vi "AO_2Chan.vi"() -> ()   [LabVIEW 2021]
doc: "This example demonstrates how to generate a user-defined voltage using the analog output of a DAQ device."
uses:
  <vilib>/Utility/error.llb/DialogType.ctl
  <vilib>/DAQmx/write.llb/DAQmx Write (Analog 1D DBL NChan 1Samp).vi
  <vilib>/DAQmx/create/channels.llb/DAQmx Create Channel (AO-Voltage-Basic).vi
  <vilib>/DAQmx/miscellaneous.llb/DAQmx Fill In Error Info.vi
panel:
  out "Iteration":i32
  in  "Tab Control":enum32{"Manual", "Toggle"}(tab)
  in  "Control":enum16{"Up", "Zero", "Down"}[](array[ring])
  out "Output":dbl[](array[numeric])
  in  "Pulse Width":u32=100
  in  "Stop":bool
  in  "Max Voltage":dbl=10.0
  in  "Min Voltage":dbl=-10.0
  in  "Physical Channel(s)":tag="Dev2/ao0:1"
  # "Channel Settings"
  # "Output"
  # "The number of elements in the channel array\nmust equal the number of channels in the task."
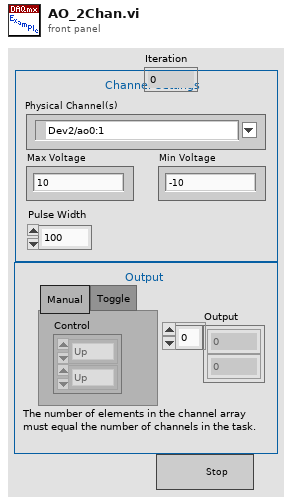
[diagram p1: front panel]
types:
  T1 = typedef "DialogType.ctl" = u16
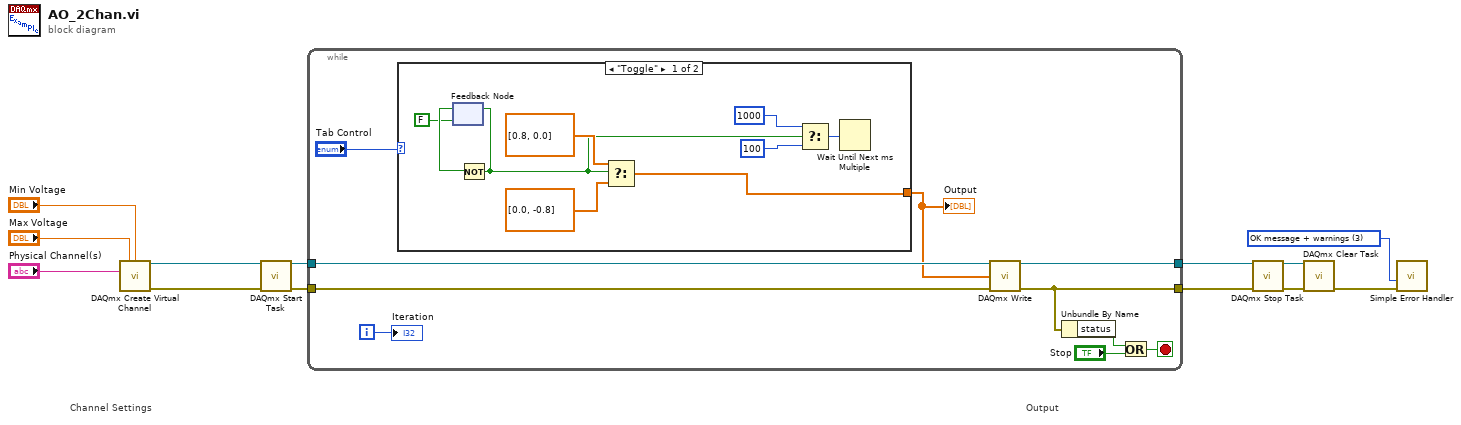
[diagram p0: block diagram]
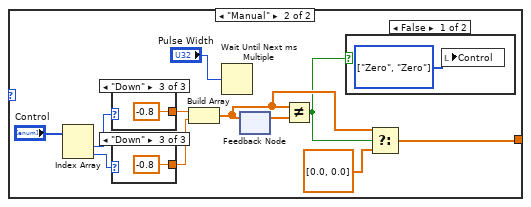
[diagram p2: hidden frame]
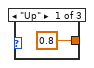
[diagram p4: hidden frame]
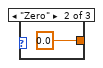
[diagram p5: hidden frame]
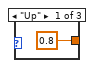
[diagram p6: hidden frame]
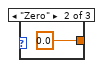
[diagram p7: hidden frame]
diagram:
  w1 = T1 3 items=["no dialog", "OK message", "continue or stop message", "OK message + warnings", "continue/stop + warnings"] ("type of dialog (OK msg:1)")
  # "Output"
  # "Channel Settings"
  n1 = call-poly <vilib>:"DAQmx Create Virtual Channel.vi"("maximum value"="Max Voltage", "minimum value"="Min Voltage", "physical channels"="Physical Channel(s)") -> ("task out"=w9:refnum<k21>, "error out"=w8:errorcluster)  [unwired: 11 in]
  n2 = call <vilib>:"DAQmx Start Task.vi"("task/channels in"=w9, "error in"=w8) -> ("task out"=w7:refnum<k21>, "error out"=w6:errorcluster)  [unwired: 12 in]
  n3 = while {
    tunnel: w7 -> [w23]
    tunnel: w6 -> [w22]
    tunnel: [w18] -> w4
    tunnel: [w21] -> w5
    i -> [w14]
    stop <- w17 stop-if-true
    n4 = case shown="\"Toggle\"" "Tab Control" {
      tunnel: [w29 w41] -> w16
      frame "Toggle" {
        n5 = feedback #1(FALSE) -> (w30:bool)
        n6 = Not(x=w30) -> (.not. x?=w25:bool)
        n7 = feedback-in #1(w25) -> ()
        n8 = Select(t=dbl[] [0.8, 0.0] ("f"), s=w25, f=dbl[] [0.0, -0.8]) -> (s? t:f=w29:dbl[])
        n9 = Select(t=u32 1000 ("Pulse Width"), s=w25, f=u32 100 ("Pulse Width")) -> (s? t:f=w28:u32)
        n10 = Wait Until Next ms Multiple(millisecond multiple=w28) -> ()  [unwired: 1 out]
      }
      frame "Manual" {
        n11 = Index Array(array="Control") -> (element #1=w39:enum16{"Up", "Zero", "Down"}, element #2=w37:enum16{"Up", "Zero", "Down"})  [unwired: 2 in]
        n12 = case shown="\"Down\"" w39 {
          tunnel: [0.8 0.0 -0.8] -> w38
          frame "Up" {
          }
          frame "Zero" {
          }
          frame "Down" {
          }
        }
        n13 = case shown="\"Down\"" w37 {
          tunnel: [0.8 0.0 -0.8] -> w36
          frame "Up" {
          }
          frame "Zero" {
          }
          frame "Down" {
          }
        }
        n14 = Build Array(w38, w36) -> (w35:dbl[])
        n15 = Wait Until Next ms Multiple(millisecond multiple="Pulse Width") -> ()  [unwired: 1 out]
        n16 = feedback #2() -> (w43:dbl[])  [unwired: 1 in]
        n17 = feedback-in #2(w35) -> ()
        n18 = Not Equal?(x=w35, y=w43) -> (x != y?=w34:bool)
        n19 = case shown="False" w34 {
          frame False {
            w44 = enum16{"Up", "Zero", "Down"}[] [enum."Zero", enum."Zero"] items=["Up", "Zero", "Down"] ("Control")
            n20 = local write "Control"(w44) -> ()
          }
          frame True {
          }
        }
        n21 = Select(t=w35, s=w34, f=dbl[] [0.0, 0.0]) -> (s? t:f=w41:dbl[])
      }
    }
    "Output" <- w16
    n22 = call-poly <vilib>:"DAQmx Write.vi"("task/channels in"=w23, "data"=w16, "error in"=w22) -> ("task out"=w21:refnum<k21>, "error out"=w18:errorcluster)  [unwired: 10 in, 1 out]
    n23 = Unbundle By Name(w18) -> ("status"=w20:bool)
    n24 = Or(x=w20, y="Stop") -> (x .or. y?=w17:bool)
    "Iteration" <- w14
  }
  n25 = call <vilib>:"DAQmx Stop Task.vi"("task/channels in"=w5, "error in"=w4) -> ("task out"=w3:refnum<k21>, "error out"=w2:errorcluster)  [unwired: 12 in]
  n26 = call <vilib>:"DAQmx Clear Task.vi"("task in"=w3, "error in"=w2) -> ("error out"=w13:errorcluster)  [unwired: 13 in]
  n27 = call <vilib>:"Simple Error Handler.vi"("type of dialog (OK msg:1)"=w1, "error in (no error)"=w13) -> ()  [unwired: 3 in, 5 out]
